vi "onListenForNewConnection.vi"(8 "error in (no error)":errorcluster, 9 "timeout (ms)":i32=1, 11 "Listener":refnum<class "WebsocketsConnection.lvclass">) -> (0 "error out":errorcluster, 1 "New connection":bool, 2 "timed out":bool, 3 "New Connection":refnum<class "Connection.lvclass">)   [LabVIEW 2013, in "MQTT_Websockets.lvlib" / "WebsocketsConnection.lvclass"]
uses:
  WebsocketsConnection.lvclass
  <vilib>/LabVIEW Open Source Project/MQTT Connection/MQTT_Connection/Connection/Connection.lvclass
  WebsocketsConnection.lvclass/WebsocketsConnection.ctl
  <vilib>/MediaMongrels Ltd/WebSockets/WebSockets/WebSocket Server/WebSocket Server.lvclass
  <vilib>/MediaMongrels Ltd/WebSockets/Sockets/VISA TCP Socket/VISA TCP.lvclass
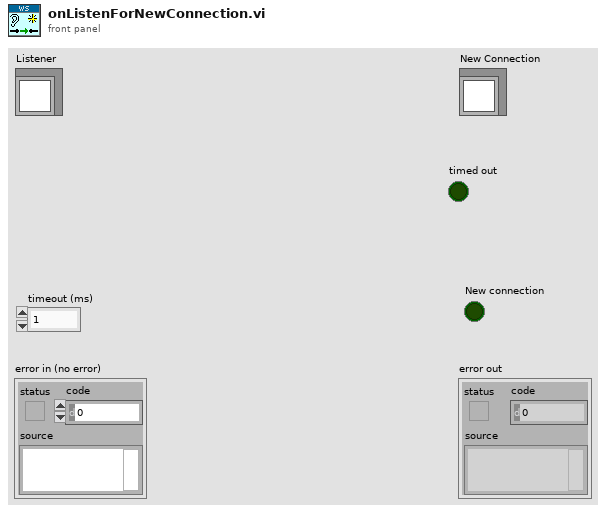
[diagram p1: front panel]
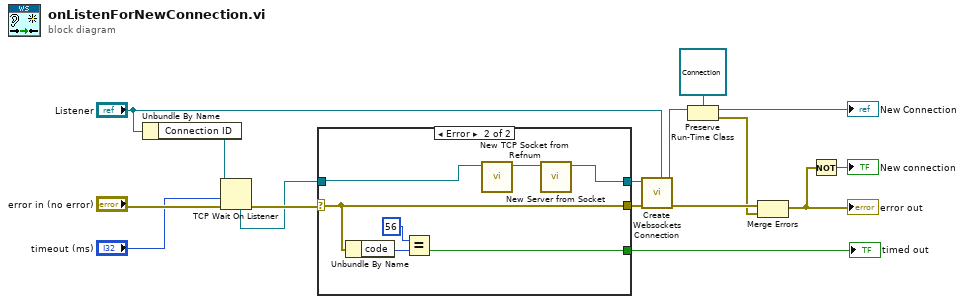
[diagram p0: block diagram]
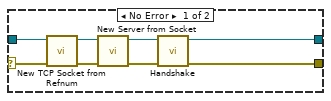
[diagram p2: hidden frame]
diagram:
  n1 = Unbundle By Name("Listener") -> ("Connection ID"=w16:refnum<k5>)
  n2 = TCP Wait On Listener(8:"error in (no error)", 9:"timeout (ms)", 11:w16) -> (0:w11:errorcluster, 4:w6:refnum<k5>)  [unwired: 1 in, 3 out]
  n3 = case shown="Error" w11 {
    selector: w11 -> [w18 w31]
    tunnel: [w22 w25] -> w14
    tunnel: [w19 w31] -> w13
    tunnel: w6 -> [w17 w27]
    tunnel: [_ w28] -> w5
    frame No Error {
      n4 = call <vilib>:"New TCP Socket from Refnum.vi"("error in (no error)"=w18, "TCP Network Connection Refnum"=w17) -> ("error out"=w21:errorcluster, "VISA TCP out"=w24:refnum<class "VISA TCP.lvclass">)  [unwired: 8 in]
      n5 = call <vilib>:"New Server from Socket.vi"("error in (no error)"=w21, "Socket"=w24) -> ("error out"=w20:errorcluster, "WebSocket Server out"=w23:refnum<class "WebSocket Server.lvclass">)  [unwired: 8 in]
      n6 = call-dynamic "Handshake.vi"("error in (no error)"=w20, "WebSocket Connection in"=w23) -> ("error out"=w19:errorcluster, "WebSocket Connection out"=w22:refnum<class "WebSocket Server.lvclass">)  [unwired: 8 in]
    }
    frame Error {
      n7 = Unbundle By Name(w31) -> ("code"=w30:i32)
      n8 = Equal?(x=56, y=w30) -> (x = y?=w28:bool)
      n9 = call <vilib>:"New TCP Socket from Refnum.vi"("TCP Network Connection Refnum"=w27) -> ("VISA TCP out"=w26:refnum<class "VISA TCP.lvclass">)  [unwired: 9 in, 1 out]
      n10 = call <vilib>:"New Server from Socket.vi"("Socket"=w26) -> ("WebSocket Server out"=w25:refnum<class "WebSocket Server.lvclass">)  [unwired: 9 in, 1 out]
    }
  }
  "timed out" <- w5
  n11 = call "Create Websockets Connection.vi"("WSConnection in"="Listener", "error in (no error)"=w13, "WebSocket"=w14) -> ("error out"=w3:errorcluster, "WSConnection"=w9:refnum<class "WebsocketsConnection.lvclass">)  [unwired: 7 in]
  n12 = Preserve Run-Time Class(object in=w9, 2:refnum<class "Connection.lvclass"> refnum ("New Connection")) -> (object out=→"New Connection":refnum<class "Connection.lvclass">, error out=w2:errorcluster)  [unwired: 1 in]
  n13 = Merge Errors(w3, w2) -> (w1:errorcluster)
  "error out" <- w1
  n14 = Not(x=w1) -> (.not. x?=→"New connection":bool)
